vi "HB_WriteToLog.vi"(8 "error in (no error)":errorcluster, 10 "Log string":string, 11 "HBDevRef":T1) -> (0 "error out":errorcluster, 3 "HBDevRef":T1)   [LabVIEW 2016]
doc: "Logs the specified string to the currently opened file on the SD card. If no file has been opened, the specified string will not be logged. The length of the string must be less than 246 characters or else no data will be logged."
uses:
  <vilib>/Rock Robotics/WPI/SerialPort/WPI_SerialPortRef.ctl
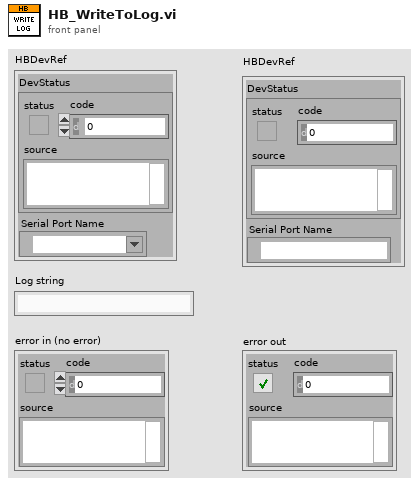
[diagram p1: front panel]
types:
  T1 = typedef "WPI_SerialPortRef.ctl" = cluster{"DevStatus":errorcluster, "Serial Port Name":refnum<visa-resource-name>}
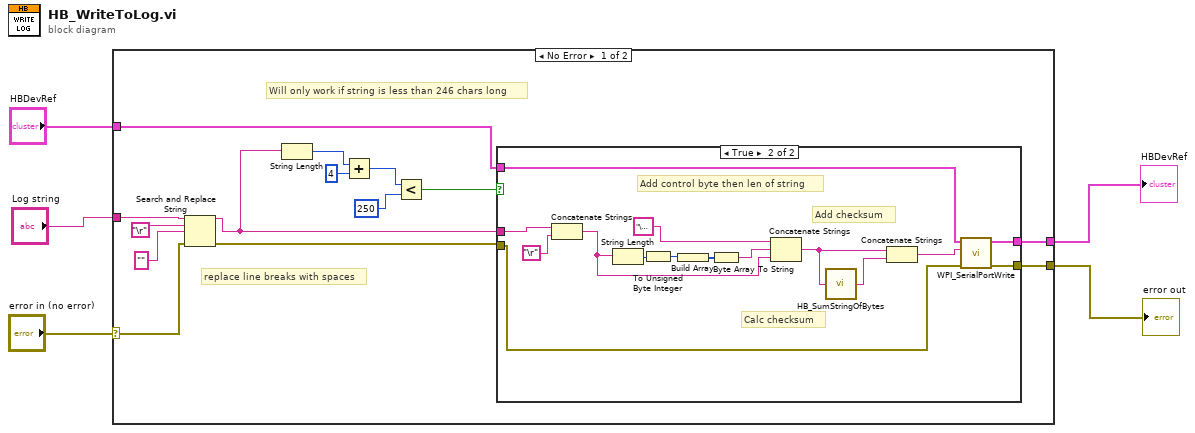
[diagram p0: block diagram]
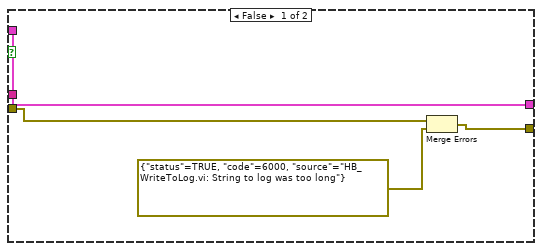
[diagram p2: hidden frame]
diagram:
  n1 = case shown="No Error" "error in (no error)" {
    selector: "error in (no error)" -> [w6 w40]
    tunnel: "Log string" -> [w18 _]
    tunnel: "HBDevRef" -> [w9 w39]
    tunnel: [w8 w39] -> w3
    tunnel: [w7 w40] -> w2
    frame No Error {
      # "Will only work if string is less than 246 chars long"
      # "replace line breaks with spaces"
      n2 = Search and Replace String(input string=w18, search string="\r", replace string="" ("replace string (\"\")"), error in=w6) -> (result string=w12:string, error out=w11:errorcluster)  [unwired: 4 in, 2 out]
      n3 = String Length(string=w12) -> (length=w14:i32)
      n4 = Add(x=w14, y=4) -> (x+y=w16:i32)
      n5 = Less?(x=w16, y=250) -> (x < y?=w13:bool)
      n6 = case shown="True" w13 {
        tunnel: w12 -> [_ w27]
        tunnel: w11 -> [w21 w26]
        tunnel: [w20 w30] -> w8
        tunnel: [w22 w29] -> w7
        tunnel: w9 -> [w20 w28]
        frame False {
          n7 = Merge Errors(w21, errorcluster {"status"=TRUE, "code"=6000, "source"="HB_WriteToLog.vi: String to log was too long"} ("error out")) -> (w22:errorcluster)
        }
        frame True {
          # "Add checksum"
          # "Add control byte then len of string"
          # "Calc checksum"
          n8 = Concatenate Strings(w27, "\r") -> (w33:string)
          n9 = String Length(string=w33) -> (length=w35:i32)
          n10 = To Unsigned Byte Integer(number=w35) -> (unsigned 8bit integer=w34:u8)
          n11 = Build Array(w34) -> (w38:u8[])
          n12 = Byte Array To String(unsigned byte array=w38) -> (string=w37:string)
          n13 = Concatenate Strings("\u0001", w37, w33) -> (w24:string)
          n14 = call <vilib>:"HB_SumStringOfBytes.vi"("String Of Bytes"=w24) -> ("Sum as String"=w25:string)
          n15 = Concatenate Strings(w24, w25) -> (w31:string)
          n16 = call <vilib>:"WPI_SerialPortWrite.vi"("error in (no error)"=w26, "Buffer"=w31, "SerialPortRef"=w28) -> ("error out"=w29:errorcluster, "SerialPortRef"=w30:T1)  [unwired: 6 in, 1 out]
        }
      }
    }
    frame Error {
    }
  }
  "HBDevRef" <- w3
  "error out" <- w2
